vi "DAQmx Create Channel (TEDS-AI-Voltage-Custom with Excitation).vi"(0 "task in":refnum<k21>, 1 "maximum value":dbl=10.0 format="%0.2f", 2 "minimum value":dbl=-10.0 format="%0.2f", 3 "input terminal configuration":i32(ring)=-1 items=["default"=-1, "RSE"=10083, "NRSE"=10078, "Differential"=10106, "Pseudodifferential"=12529], 5 "physical channels":tag, 7 "name to assign":string, 9 "units":i32(ring)=12516 items=["From TEDS"=12516, "From Custom Scale"=10065], 10 "voltage excitation value":dbl format="%.6f", 11 "error in":errorcluster, 12 "custom scale name":tag, 13 "voltage excitation source":i32(ring)=10200 items=["Internal"=10200, "External"=10167, "None"=10230]) -> (4 "task out":refnum<k21>, 15 "error out":errorcluster)   [LabVIEW 2013]
doc: "Creates channel(s) to measure voltage. Use this instance for custom sensors that require excitation. You can use the excitation to scale the measurement. You must configure the physical channel(s) with TEDS information to use this VI."
uses:
  nilvaiu.dll
panel:
  # "input limits"
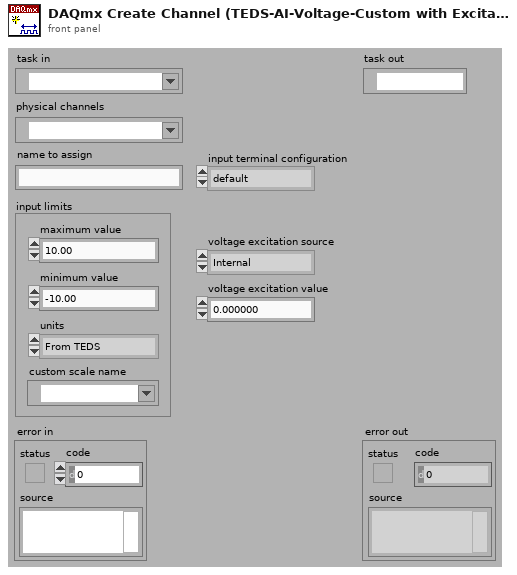
[diagram p1: front panel]
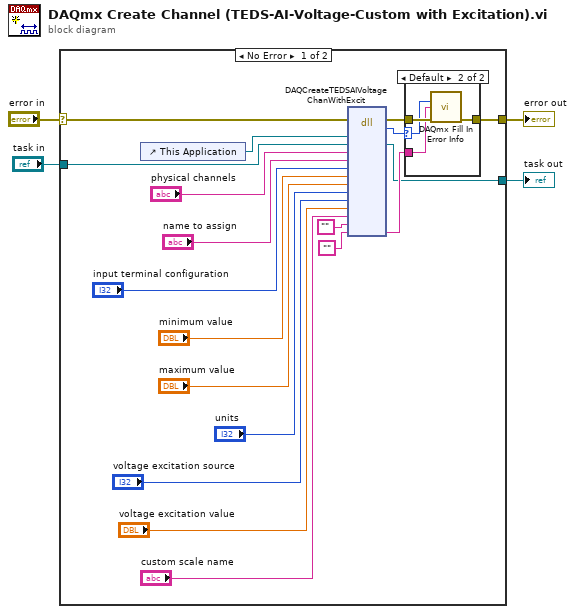
[diagram p0: block diagram]
diagram:
  n1 = case shown="No Error" "error in" {
    selector: "error in" -> [w8 w29]
    tunnel: "task in" -> [w10 w30]
    tunnel: [w9 w30] -> w3
    tunnel: [w7 w29] -> w1
    frame No Error {
      n2 = control-ref of="This Application"() -> (w11:refnum<vi>)
      n3 = dll-call lib="nilvaiu.*" fn="DAQCreateTEDSAIVoltageChanWithExcit"(error in=w8, "lvAppRef"=w11, "refObjPtr"=w10, "physicalChannelName"="physical channels", "channelNameIn"="name to assign", "terminalConfig"="input terminal configuration", "minVal"="minimum value", "maxVal"="maximum value", "units"="units", "excitSource"="voltage excitation source", "excitVal"="voltage excitation value", "customScaleName"="custom scale name", "channelNamesOut"="", "extendedErrorInfo"="") -> (error out=w23:errorcluster, "return type"=w22:i32, "refObjPtr"=w9:refnum<k21>, "extendedErrorInfo"=w21:string)  [unwired: 13 in, 1 out]
      n4 = case shown="Default" w22 {
        selector: w22 -> [_ w26]
        tunnel: w23 -> [w24 w28]
        tunnel: [w24 w27] -> w7
        tunnel: w21 -> [_ w25]
        frame 0 {
        }
        frame Default {
          n5 = call "DAQmx Fill In Error Info.vi"("status code"=w26, "extended error info"=w25, "error in"=w28) -> ("error out"=w27:errorcluster)  [unwired: 1 in, 11 out]
        }
      }
    }
    frame Error {
    }
  }
  "task out" <- w3
  "error out" <- w1
